vi "Initialize Display Format.vi"(8 "error in (no error)":errorcluster, 11 "Numeric Data Type in":refnum<class "Numeric Data Type.lvclass">) -> (0 "error out":errorcluster, 3 "Numeric Data Type (dup)":refnum<class "Numeric Data Type.lvclass">)   [LabVIEW 2018, in "Numeric Data Type.lvclass"]
uses:
  Numeric Data Type.lvclass
  Numeric Data Type.lvclass/Numeric Data Type.ctl
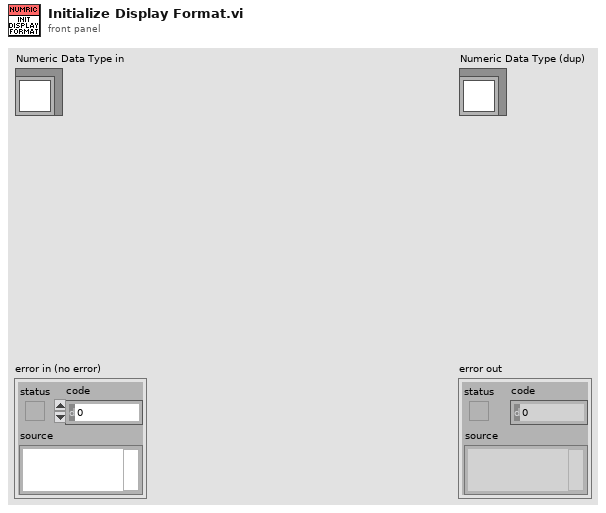
[diagram p1: front panel]
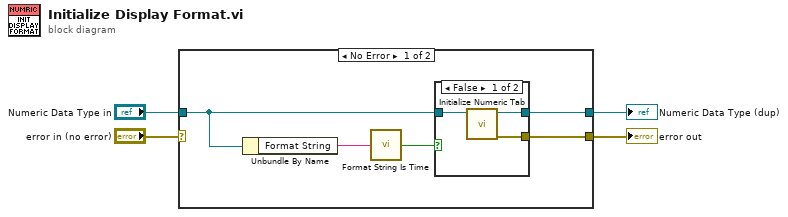
[diagram p0: block diagram]
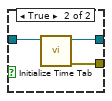
[diagram p2: hidden frame]
diagram:
  n1 = case shown="No Error" "error in (no error)" {
    selector: "error in (no error)" -> [_ w17]
    tunnel: [w5 w17] -> w3
    tunnel: [w6 w16] -> w1
    tunnel: "Numeric Data Type in" -> [w8 w16]
    frame No Error {
      n2 = Unbundle By Name(w8) -> ("Format String"=w9:string)
      n3 = call "Format String Is Time.vi"("Format String"=w9) -> ("Time?"=w7:bool)
      n4 = case shown="False" w7 {
        tunnel: w8 -> [w12 w15]
        tunnel: [w11 w14] -> w6
        tunnel: [w10 w13] -> w5
        frame False {
          n5 = call "Initialize Numeric Tab.vi"("Numeric Data Type in"=w12) -> ("error out"=w10:errorcluster, "Numeric Data Type (dub)"=w11:refnum<class "Numeric Data Type.lvclass">)  [unwired: 9 in]
        }
        frame True {
          n6 = call "Initialize Time Tab.vi"("Numeric Data Type in"=w15) -> ("error out"=w13:errorcluster, "Numeric Data Type (dub)"=w14:refnum<class "Numeric Data Type.lvclass">)  [unwired: 9 in]
        }
      }
    }
    frame Error {
    }
  }
  "error out" <- w3
  "Numeric Data Type (dup)" <- w1
